vi "PreprocessTimeoutResponse.vi"(8 "error in (no error)":errorcluster, 10 "response in":T1, 11 "BaseDriver In":refnum<class "BaseDriver.lvclass">) -> (0 "error out":errorcluster, 2 "response out":T1, 3 "BaseDriver Out":refnum<class "BaseDriver.lvclass">)   [LabVIEW 2025, in "BaseDriver.lvclass"]
doc: "Preform any processing of a generated timeout response before sending i to the caller"
uses:
  BaseDriver.lvclass
  response.ctl
  driver_status.ctl
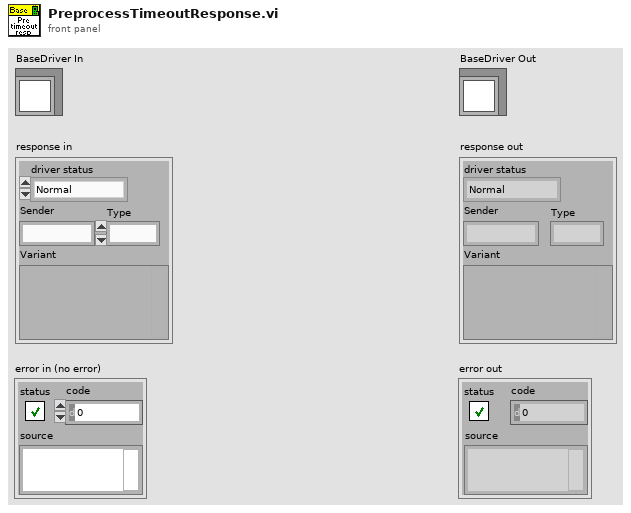
[diagram p1: front panel]
types:
  T1 = typedef "response.ctl" = cluster{"driver status":T2, "Sender":string, "Type":i32, "Variant":variant}
  T2 = typedef "driver_status.ctl" = enum16{"Normal", "Startup", "Connection lost", "Reconnected", "Timeout", "Idle", "Busy"}
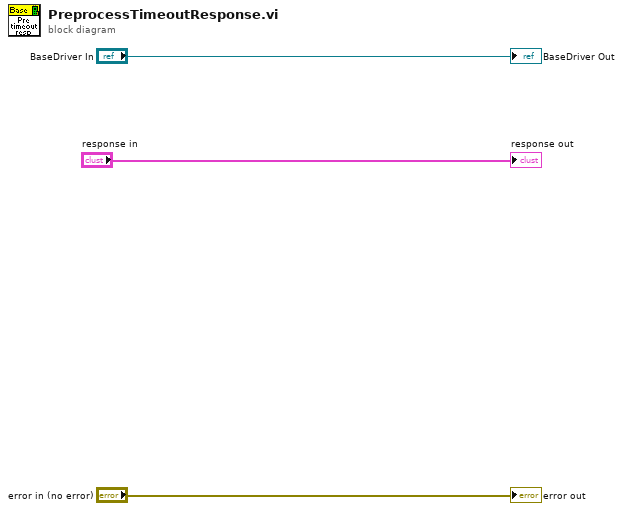
[diagram p0: block diagram]
diagram:
  "error out" <- "error in (no error)"
  "BaseDriver Out" <- "BaseDriver In"
  "response out" <- "response in"
